vi "tsapp_set_lin_channel_count.vi"(8 "error in (no error)":errorcluster, 10 "Aount":i32, 11 "Path":path) -> (0 "error out":errorcluster, 2 "return":i32, 3 "Path output":path)   [LabVIEW 2014]
doc: "Function Introduction :\nSet the number of CAN channels used by the application. You can directly access it through the TSMaster interface\nCompleted.\nCall location :\nBefore mapping LIN channels, users can allocate the necessary resources based on the application's requirements\nThe number of LIN channels.\ninput parameter :\nACount: The number of LIN channels that need to be set\nReturn value :\n==0: Setting successful\nOther: Failed, query error type based on error code"
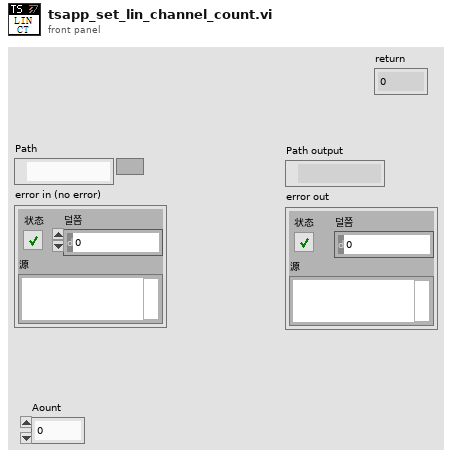
[diagram p1: front panel]
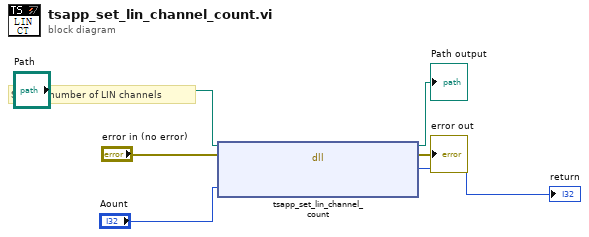
[diagram p0: block diagram]
diagram:
  # "Set the number of LIN channels"
  n1 = dll-call lib="PTH2@abs EDemo同星TSCAN_V1.4_20220301ConfigTSMaster.dll" fn="tsapp_set_lin_channel_count"(path in="Path", error in="error in (no error)", "Aount"="Aount") -> (path out=→"Path output":path, error out=→"error out":errorcluster, "tsapp_set_lin_channel_count"=→"return":i32)  [unwired: 2 in]
